vi "Get Cost.vi"(8 "error in (no error)":errorcluster, 11 "Beverage in":refnum<class "Beverage.lvclass">) -> (0 "error out":errorcluster, 2 "Cost":dbl, 3 "Beverage out":refnum<class "Beverage.lvclass">)   [LabVIEW 2020, in "Beverage.lvclass"]
doc: "Return the <b>Cost</b> of a Beverage."
uses:
  Beverage.lvclass
  Beverage.lvclass/Beverage.ctl
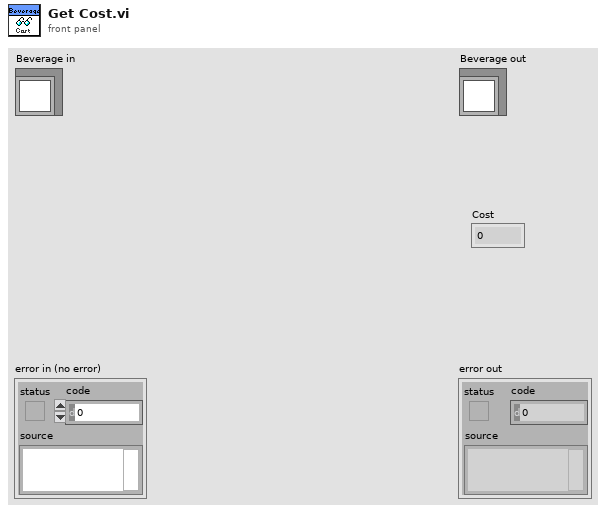
[diagram p1: front panel]
types:
  T1 = typedef "Beverage.lvclass/Options.ctl" = enum16{"<None>", "Milk", "Mocha", "Soy", "Whip"}
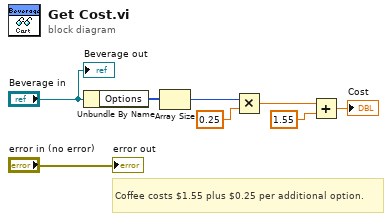
[diagram p0: block diagram]
diagram:
  # "Coffee costs $1.55 plus $0.25 per additional option."
  n1 = Unbundle By Name("Beverage in") -> ("Options"=w6:T1[])
  n2 = Array Size(array=w6) -> (size(s)=w5:i32)
  n3 = Multiply(x=w5, y=0.25) -> (x*y=w3:dbl)
  n4 = Add(x=w3, y=1.55) -> (x+y=→"Cost":dbl)
  "error out" <- "error in (no error)"
  "Beverage out" <- "Beverage in"
